vi "Create Phrase ASCII or Unicode.vi"(0 "Character type":T1=enum."ASCII", 7 "Text":string, 11 "error in (no error)":errorcluster) -> (8 "Phrase refnum":refnum<k24>, 10 "Char U16 [ ]":u16[](array[numeric]) format="%04x", 15 "error out":errorcluster)   [LabVIEW 2020, in "Exaprom PDF.lvlib"]
doc: "Developed by Jean-Marc Simard\nCopyright © 2012, Exaprom Inc.\nAll rights reserved.\nLicense: BSD\n\nWith iTextSharp 4.1.6 (http://itextsharp.sourceforge.net)\nunder Mozilla Public License Version 1.1\n(http://www.mozilla.org/MPL/MPL-1.1.html)"
uses:
  <userlib>/labview-PDF-writer-master/Exaprom PDF.lvlib
  <userlib>/labview-PDF-writer-master/Controls/Text Controls/Unicode/Type and run direction.ctl
  C:/Program Files (x86)/National Instruments/LabVIEW 2020/user.lib/labview-PDF-writer-master/DLL/itextsharp.dll
  DLL/itextsharp.dll
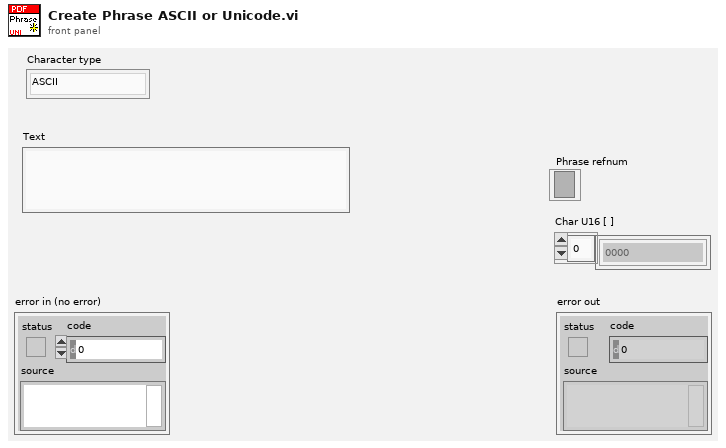
[diagram p1: front panel]
types:
  T1 = typedef "Exaprom PDF.lvlib/Type and run direction.ctl" = enum16{"Select", "ASCII", "UTF-16", "UTF-16 (default)", "UTF-16 (LTR)", "UTF-16 (RTL)"}
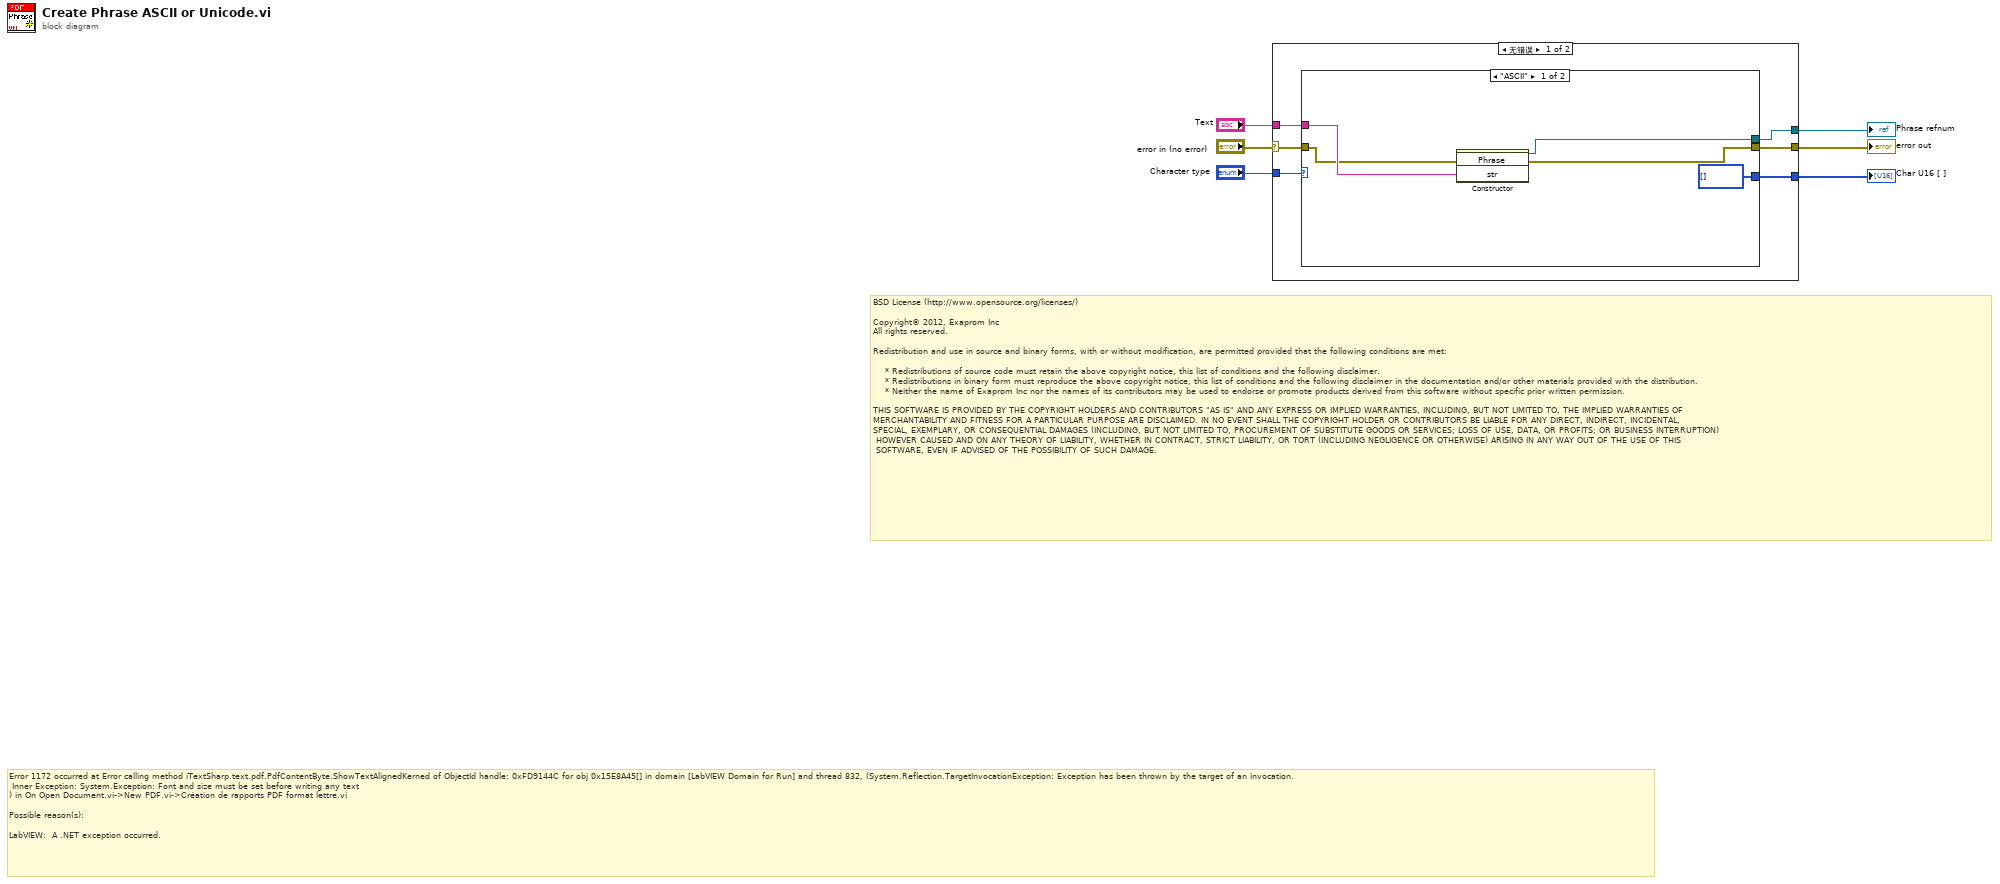
[diagram p0: block diagram]
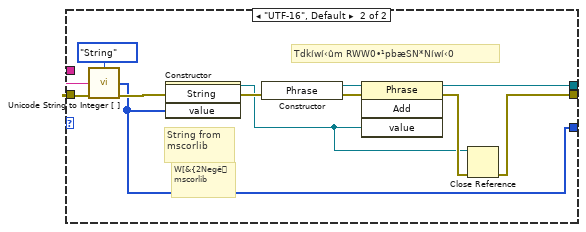
[diagram p2: hidden frame]
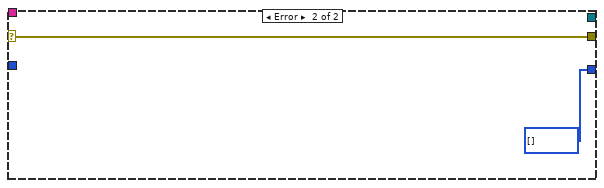
[diagram p3: hidden frame]
diagram:
  # "Error 1172 occurred at Error calling method iTextSharp.text.pdf.PdfContentByte.ShowTextAlignedKerned of ObjectId handle: 0xFD9144C for obj 0x15E8A45[] in domain [LabVIEW Domain for Run] and thread 832, (System.Reflection.TargetInvocationException: Exception has been thrown by the target of an invocation.\n\tInner Exception: System.Exception: Font and size must be set before writing any text\n) in On Open Document.vi->New PDF.vi->Création de rapports PDF format lettre.vi\n\nPossible reason(s):\n\nLabVIEW:  A .NET exception occurred."
  # "BSD License (http://www.opensource.org/licenses/)\n\nCopyright© 2012, Exaprom Inc\nAll rights reserved.\n\nRedistribution and use in source and binary forms, with or without modification, are permitted provided that the following conditions are met:\n\n    * Redistributions of source code must retain the above copyright notice, this list of conditions and the following disclaimer.\n    * Redistributions in binary form must reproduce the above copyright notice, this list of conditions and the following disclaimer in the documentation and/or other materials provided with the distribution.\n    * Neither the name of Exaprom Inc nor the names of its contributors may be used to endorse or promote products derived from this software without specific prior written permission.\n\nTHIS SOFTWARE IS PROVIDED BY THE COPYRIGHT HOLDERS AND CONTRIBUTORS \"AS IS\" AND ANY EXPRESS OR IMPLIED WARRANTIES, INCLUDING, BUT NOT LIMITED TO, THE IMPLIED WARRANTIES OF \nMERCHANTABILITY AND FITNESS FOR A PARTICULAR PURPOSE ARE DISCLAIMED. IN NO EVENT SHALL THE COPYRIGHT HOLDER OR CONTRIBUTORS BE LIABLE FOR ANY DIRECT, INDIRECT, INCIDENTAL,\nSPECIAL, EXEMPLARY, OR CONSEQUENTIAL DAMAGES (INCLUDING, BUT NOT LIMITED TO, PROCUREMENT OF SUBSTITUTE GOODS OR SERVICES; LOSS OF USE, DATA, OR PROFITS; OR BUSINESS INTERRUPTION)\n HOWEVER CAUSED AND ON ANY THEORY OF LIABILITY, WHETHER IN CONTRACT, STRICT LIABILITY, OR TORT (INCLUDING NEGLIGENCE OR OTHERWISE) ARISING IN ANY WAY OUT OF THE USE OF THIS\n SOFTWARE, EVEN IF ADVISED OF THE POSSIBILITY OF SUCH DAMAGE."
  n1 = case shown="无错误" "error in (no error)" {
    selector: "error in (no error)" -> [w10 w31]
    tunnel: [w11 w31] -> w6
    tunnel: "Character type" -> [w12 _]
    tunnel: [w9 _] -> w3
    tunnel: "Text" -> [w8 _]
    tunnel: [w7 u16[] [] ("Char U16 [ ]")] -> w1
    frame No Error {
      n2 = case shown="\"ASCII\"" w12 {
        tunnel: w10 -> [w13 w22]
        tunnel: [w16 w28] -> w9
        tunnel: [w17 w27] -> w11
        tunnel: w8 -> [w14 w20]
        tunnel: [u16[] [] ("Char U16 [ ]") w18] -> w7
        frame "ASCII" {
          n3 = constructor class="Phrase"(error in=w13, "str"=w14) -> (reference out=w16:refnum<k24>, error out=w17:errorcluster)  [unwired: 2 in, 2 out]
        }
        frame "UTF-16", Default {
          # "Tdkíwí‹ûm RWW0•¹pbæSN*Níwí‹0"
          # "W[&{2Negê\nmscorlib"
          # "String from\nmscorlib"
          n4 = call <userlib>:"Unicode String to Integer [ ].vi"("From"=enum16{"String", "U16 [ ]"}."String", "Unicode String"=w20, "error in (no error)"=w22) -> ("Char U16 [ ]"=w18:u16[], "error duplicate"=w21:errorcluster)  [unwired: 10 in, 1 out]
          n5 = constructor class="String" ("Constructor Node")(error in=w21, "value"=w18) -> (reference out=w25:refnum<k24>, error out=w29:errorcluster)  [unwired: 2 in, 2 out]
          n6 = constructor class="Phrase"(error in=w29) -> (reference out=w24:refnum<k24>, error out=w23:errorcluster)  [unwired: 2 in, 1 out]
          n7 = invoke class="Phrase" method="Add"(reference=w24, error in=w23, "value"=w25) -> (reference out=w28:refnum<k24>, error out=w26:errorcluster)  [unwired: 1 in, 2 out]
          n8 = Close Reference(reference=w25, error in (no error)=w26) -> (error out=w27:errorcluster)
        }
      }
    }
    frame Error {
    }
  }
  "error out" <- w6
  "Phrase refnum" <- w3
  "Char U16 [ ]" <- w1
